vi "Reset Device Core.vi"(8 "error in (no error)":errorcluster, 11 "CS++Motor in":refnum<class "CS++Motor.lvclass">) -> (0 "error out":errorcluster, 3 "CS++Motor out":refnum<class "CS++Motor.lvclass">)   [LabVIEW 2015, in "CS++Motor.lvlib" / "CS++Motor.lvclass"]
doc: "Perform reset of device."
uses:
  CS++Motor.lvclass
  CSPP_Core/Classes/CS++ProcessVariables/ProcessVariable/PV.lvclass
  PV-Enum-n.ctl
  CS++Motor.lvclass/CS++Motor.ctl
  CSPP_Core/Classes/CS++ProcessVariables/ProcessVariable/PV.lvclass/PV.ctl
  CSPP_Core/Classes/CS++ProcessVariables/ProcessVariable/Write Data.vi
  CSPP_Core/Classes/CS++ProcessVariables/ProcessVariable/Write Timestamp.vi
  CSPP_Core/Classes/CS++ProcessVariables/ProcessVariable/Write Quality.vi
  CSPP_Core/Classes/CS++ProcessVariables/ProcessVariable/Write status.vi
  CSPP_Core/Actors/CS++DeviceActor/CS++DeviceActor.lvclass
  CSPP_Core/Classes/CS++ProcessVariables/PVConnection/PVConnection.lvclass
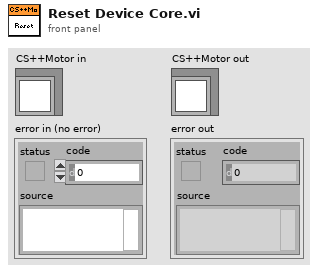
[diagram p1: front panel]
types:
  T1 = typedef "CS++Motor.lvlib/CS++Motor.lvclass/PV-Enum-n.ctl" = enum16{"PhysicalName", "unit", "ActPosition", "SetPosition", "RawSetPosition", "StartVelocity", "StopVelocity", "Acceleration", "RangeMin", "RangeMax", "Scaling", "ScalingOffset", "RangeRefError", "LogicalPositionArray", "NoOfCommands"}
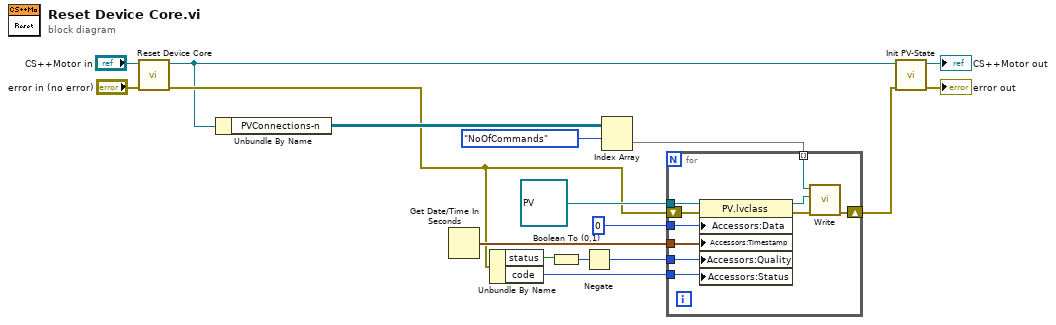
[diagram p0: block diagram]
diagram:
  n1 = call-parent "Reset Device Core.vi"("error in (no error)"="error in (no error)", "CS++DeviceActor in"="CS++Motor in") -> ("error out"=w5:errorcluster, "CS++DeviceActor out"=w4:refnum<class "CS++Motor.lvclass">)  [unwired: 8 in]
  n2 = Unbundle By Name(w4) -> ("PVConnections-n"=w7:refnum<class "PVConnection.lvclass">[][])
  n3 = Get Date/Time In Seconds() -> (seconds since 1Jan1904=w11:timestamp)
  n4 = Unbundle By Name(w5) -> ("status"=w12:bool, "code"=w14:i32)
  n5 = Boolean To (0,1)(Boolean=w12) -> (0, 1=w13:i16)
  n6 = Negate(x=w13) -> (-x=w15:i16)
  n7 = Index Array(array=w7, index (row)=PV-Enum-n."NoOfCommands" ("PV-Enum-n")) -> (element=w6:refnum<class "PVConnection.lvclass">[])  [unwired: 1 in]
  n8 = for {
    tunnel: w15 -> [w27]
    tunnel: w14 -> [w26]
    tunnel: w11 -> [w25]
    tunnel: refnum<class "PV.lvclass"> refnum ("PV") -> [w21]
    tunnel: 0 -> [w19]
    shift-right: [w23] -> w2
    shift-left: w5 -> [w20]
    tunnel: w6 -> [w18] mode=indexing
    n9 = property class="PV.lvclass"(reference=w21, error in=w20, "Accessors:Data"=w19, "Accessors:Timestamp"=w25, "Accessors:Quality"=w27, "Accessors:Status"=w26) -> (reference out=w22:refnum<class "PV.lvclass">, error out=w24:errorcluster)
    n10 = call "Write.vi"("error in (no error)"=w24, "PV"=w22, "PVConnection in"=w18) -> ("error out"=w23:errorcluster)  [unwired: 7 in, 1 out]
  }
  n11 = call "Init PV-State.vi"("error in (no error)"=w2, "CS++Motor in"=w4) -> ("error out"=→"error out":errorcluster, "CS++Motor out"=→"CS++Motor out":refnum<class "CS++Motor.lvclass">)  [unwired: 8 in]
